vi "serialization tests.vi"() -> ()   [LabVIEW 2013, in "FPGA Module tests.lvlib"]
doc: "Tests the 'To String' and 'From String' methods of the Module's configuration class and ensures they are compatible."
uses:
  FPGA Module tests.lvlib
  module/configuration/FPGA Module configuration.lvclass
  module/configuration/FPGA Module configuration.lvclass/FPGA Module configuration.ctl
  <vilib>/NI/Tag Bus Module Framework/channel/TBM channel.lvclass
panel:
  out "lines equal 2":bool
  out "lines equal":bool
  out "modules equal":bool
  out "channels equal":bool
  out "no error":errorcluster
  out "no error":errorcluster
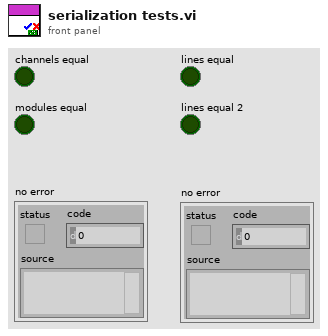
[diagram p1: front panel]
types:
  T1 = typedef "FPGA Module configuration.lvclass/Line.ctl" = cluster{"channel":refnum<class "TBM channel.lvclass">}
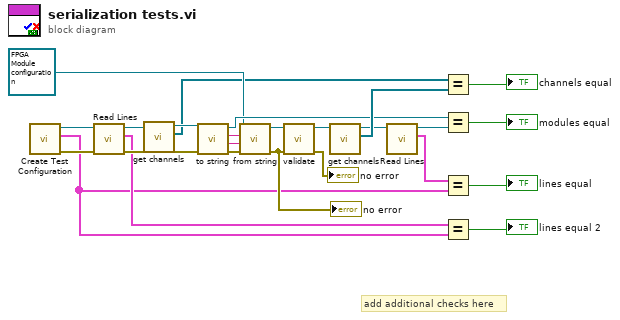
[diagram p0: block diagram]
diagram:
  # "add additional checks here"
  n1 = call "Create Test Configuration.vi"() -> ("error out"=w7:errorcluster, "Line Array"=w1:T1[], "Module Configuration"=w5:refnum<class "FPGA Module configuration.lvclass">)  [unwired: 6 in, 3 out]
  n2 = call "Read Lines.vi"("error in (no error)"=w7, "FPGA Module configuration in"=w5) -> ("error out"=w6:errorcluster, "Lines"=w2:T1[], "FPGA Module configuration out"=w4:refnum<class "FPGA Module configuration.lvclass">)  [unwired: 7 in]
  n3 = call-dynamic "get channels.vi"("FPGA Module configuration in"=w4) -> ("channels"=w12:refnum<class "TBM channel.lvclass">[], "FPGA Module configuration out"=w13:refnum<class "FPGA Module configuration.lvclass">)  [unwired: 9 in]
  n4 = call-dynamic "to string.vi"("error in"=w6, "FPGA Module configuration in"=w13) -> ("error out"=w25:errorcluster, "data"=w24:string, "version"=w23:string, "FPGA Module configuration out"=w15:refnum<class "FPGA Module configuration.lvclass">)  [unwired: 6 in]
  n5 = call-dynamic "from string.vi"("error in"=w25, "data"=w24, "version"=w23, "FPGA Module configuration in"=refnum<class "FPGA Module configuration.lvclass"> refnum ("tag bus configurable plugin module configuration")) -> ("error out"=w20:errorcluster, "FPGA Module configuration out"=w22:refnum<class "FPGA Module configuration.lvclass">)  [unwired: 6 in]
  "no error" <- w20
  n6 = call-dynamic "validate.vi"("error in"=w20, "FPGA Module configuration in"=w22) -> ("error out"=→"no error":errorcluster, "FPGA Module configuration out"=w18:refnum<class "FPGA Module configuration.lvclass">)  [unwired: 8 in]
  n7 = call-dynamic "get channels.vi"("FPGA Module configuration in"=w18) -> ("channels"=w17:refnum<class "TBM channel.lvclass">[], "FPGA Module configuration out"=w11:refnum<class "FPGA Module configuration.lvclass">)  [unwired: 9 in]
  n8 = call "Read Lines.vi"("FPGA Module configuration in"=w11) -> ("Lines"=w9:T1[], "FPGA Module configuration out"=w10:refnum<class "FPGA Module configuration.lvclass">)  [unwired: 8 in, 1 out]
  n9 = Equal?(x=w12, y=w17) -> (x = y?=→"channels equal":bool)
  n10 = Equal?(x=w15, y=w10) -> (x = y?=→"modules equal":bool)
  n11 = Equal?(x=w9, y=w1) -> (x = y?=→"lines equal":bool)
  n12 = Equal?(x=w2, y=w1) -> (x = y?=→"lines equal 2":bool)
